vi "SV TDMS Write Spectrum (1 Ch).vi"(0 "tdms file":refnum<k34>, 2 "write mode":u16(ring)=1 items=["Append", "New group", "Overwrite"], 5 "group name in":string="Spectrum", 7 "channel name in":string="Channel0", 9 "spectrum":cluster{"x0":dbl, "dx":dbl, "array":dbl[]}, 11 "error in":errorcluster, 12 "component":T1=32 items=["Magnitude"=32, "Phase"=33, "Real"=34, "Imaginary"=35, "Coherence"=36, "Unknown"=99], 13 "spectrum info":T2 {"x-axis units" items=["Time (s)"=0, "Frequency-CB (Hz)"=1, "Frequency-CPB (Hz)"=1248, "Frequency-Arbitrary (Hz)"=2357, "Quefrency (s)"=2, "Revolutions (rev)"=3, "Order"=4, "Speed (RPM)"=11, "Speed (rad/s)"=21, "Index"=65535]; "weighting filter" items=["Linear", "A-weighting", "B-weighting", "C-weighting", "ITU-R 468-4", "Dolby", "CCITT", "C-message", "Wb", "Wc", "Wd", "We", "Wf", "Wh", "Wj", "Wk", "Wm", "AES17 20 kHz lowpass", "AES17 40 kHz lowpass", "AES17 20 kHz highpass", "AES17 40 kHz highpass"]; "dB reference [EU]" format="%.2f"; "engineering units" items=["custom..."=0, "V"=1, "A"=21, "C"=30, "pC"=31, "s"=32, "-"=29, "Pa"=2, "N"=20, "g"=3, "m/s^2"=4, "m/s"=5, "m"=6, "mm/s"=12, "mm"=13, "micron/s"=14, "micron"=15, "in/s^2"=7, "in/s"=8, "in"=9, "mil/s"=10, "mil"=11, "rad/s^2"=16, "rad/s"=17, "rad"=18, "deg/s^2"=26, "deg/s"=27, "deg"=28, "RPM"=22, "cycle/s^2"=23, "Hz"=24, "cycle"=25, "strain"=19]; "spectral info"."window" items=["None "=0, "Hanning"=1, "Hamming"=2, "Blackman-Harris"=3, "Exact Blackman"=4, "Blackman"=5, "Flat Top"=6, "4 Term B-Harris "=7, "7 Term B-Harris"=8, "Low Sidelobe"=9, "Force - Exponential"=10, "Gaussian"=62]}) -> (4 "tdms file out":refnum<k34>, 6 "group name out":string, 8 "channel name out":string, 15 "error out":errorcluster)   [LabVIEW 2017]
doc: "Writes data to the specified .tdms file in a format specific to the polymorphic instance. Wire data to the <B>scaled signal [EU]</B> input to determine the polymorphic instance to use or manually select the instance."
uses:
  <vilib>/addons/_NISVFA/_Shared subVIs/Controls/svc_Spectrum Info.ctl
  <vilib>/addons/_NISVFA/_Shared subVIs/Controls/svc_X-Axis Units.ctl
  <vilib>/addons/_NISVFA/_Shared subVIs/Controls/svc_Spectrum Type.ctl
  <vilib>/addons/_NISVFA/_Shared subVIs/Controls/svc_Engineering Units Text Ring.ctl
  <vilib>/addons/_NISVFA/_Shared subVIs/Controls/svc_Weighting Filter Text Ring.ctl
  <vilib>/addons/_NISVFA/_Shared subVIs/Controls/svc_Complimentary Spectrum Units.ctl
  <vilib>/addons/_NISVFA/_Shared subVIs/Controls/NI Spectrum Component.ctl
  <vilib>/addons/_NISVFA/_Shared subVIs/Controls/LV Datatypes.ctl
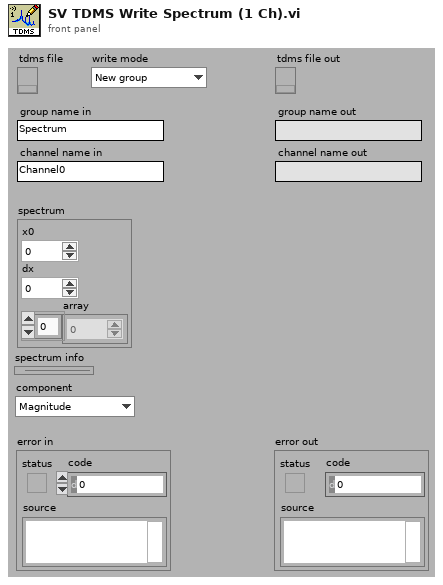
[diagram p1: front panel]
types:
  T1 = typedef "NI Spectrum Component.ctl" = u16
  T2 = typedef "svc_Spectrum Info.ctl" = cluster{"channel name":string, "description":string, "x-axis units":T3, "spectral info":cluster{"spectrum type":T4, "linear/dB":enum16{"linear", "dB"}, "window":u16, "window size":i32, "FFT size":i32}, "engineering units":T5, "custom label":string, "dB reference [EU]":dbl, "peak units":enum16{"rms", "peak", "peak-peak"}, "weighting filter":T6, "spectral density?":bool, "unit label":string, "spectrum skewed?":bool, "complimentary spectrum units":T7}
  T3 = typedef "svc_X-Axis Units.ctl" = u16
  T4 = typedef "svc_Spectrum Type.ctl" = enum16{"FFT Spectrum [complex]", "Amplitude [Magnitude]", "Power [Magnitude^2]", "Cross Spectrum [complex]", "Frequency Response [Complex]"}
  T5 = typedef "svc_Engineering Units Text Ring.ctl" = u16
  T6 = typedef "svc_Weighting Filter Text Ring.ctl" = u16
  T7 = typedef "svc_Complimentary Spectrum Units.ctl" = enum16{"none", "radians", "degrees", "cycles", "imaginary"}
  T8 = typedef "LV Datatypes.ctl" = i32
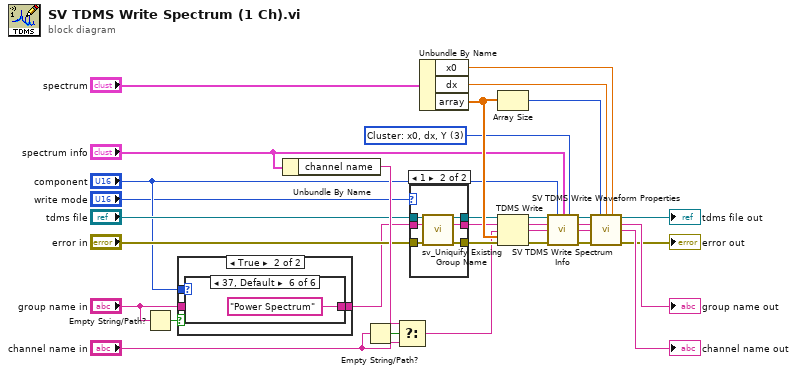
[diagram p0: block diagram]
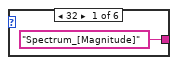
[diagram p4: hidden frame]
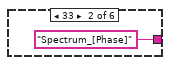
[diagram p5: hidden frame]
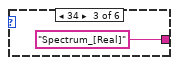
[diagram p6: hidden frame]
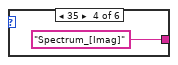
[diagram p7: hidden frame]
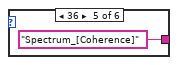
[diagram p8: hidden frame]
diagram:
  w1 = T8 3 items=["String: abc"=-2, "Boolean: True or False"=-1, "Scalar: y"=0, "Array: Y"=1, "Waveform: t0, dt, Y, variant"=2, "Cluster: x0, dx, Y"=3, "Cluster: X, Y"=4, "Waterfall"=5, "Colormap"=6] ("LabVIEW datatype")
  n1 = Empty String/Path?(string/path="group name in") -> (empty?=w21:bool)
  n2 = case shown="True" w21 {
    tunnel: "component" -> [_ w36]
    tunnel: [w34 w35] -> w22
    tunnel: "group name in" -> [w34 _]
    frame False {
    }
    frame True {
      n3 = case shown="37, Default" w36 {
        tunnel: ["Spectrum_[Magnitude]" "Spectrum_[Phase]" "Spectrum_[Real]" "Spectrum_[Imag]" "Spectrum_[Coherence]" "Power Spectrum"] -> w35
        frame 32 {
        }
        frame 33 {
        }
        frame 34 {
        }
        frame 35 {
        }
        frame 36 {
        }
        frame 37, Default {
        }
      }
    }
  }
  n4 = Unbundle By Name("spectrum info") -> ("channel name"=w31:string)
  n5 = Empty String/Path?(string/path="channel name in") -> (empty?=w28:bool)
  n6 = Select(t=w31, s=w28, f="channel name in") -> (s? t:f=w30:string)
  n7 = case shown="1" "write mode" {
    tunnel: [w43 w51] -> w32
    tunnel: [w44 w50] -> w26
    tunnel: "error in" -> [w43 w49]
    tunnel: [w45 w48] -> w23
    tunnel: w22 -> [w44 w47]
    tunnel: "tdms file" -> [w45 w46]
    frame 0, Default {
    }
    frame 1 {
      n8 = call <vilib>:"sv_Uniquify Existing Group Name.vi"("tdms file ref"=w46, "group name"=w47, "error in"=w49) -> ("tdms file out"=w48:refnum<k34>, "unique group"=w50:string, "error out"=w51:errorcluster)  [unwired: 10 in]
    }
  }
  n9 = Unbundle By Name("spectrum") -> ("x0"=w15:dbl, "dx"=w16:dbl, "array"=w33:dbl[])
  n10 = Array Size(array=w33) -> (size(s)=w17:i32)
  n11 = TDMS Write(0:w23, 5:w26, 7:w30, 9:w33, 11:w32) -> (4:w10:refnum<k34>, 6:w9:string, 8:w8:string, 15:w7:errorcluster)  [unwired: 1 in]
  n12 = call <vilib>:"SV TDMS Write Spectrum Info.vi"("tdms file"=w10, "spectrum component"="component", "spectrum info"="spectrum info", "LabVIEW datatype"=w1, "group name in"=w9, "channel name in"=w8, "error in"=w7) -> ("tdms file out"=w11:refnum<k34>, "group name out"=w12:string, "channel name out"=w13:string, "error out"=w14:errorcluster)  [unwired: 3 in, 2 out]
  n13 = call <vilib>:"SV TDMS Write Waveform Properties.vi"("tdms file"=w11, "array length"=w17, "dx"=w16, "x0"=w15, "group name"=w12, "channel name"=w13, "error in (no error)"=w14) -> ("tdms file out"=→"tdms file out":refnum<k34>, "group name out"=→"group name out":string, "channel name out"=→"channel name out":string, "error out"=→"error out":errorcluster)  [unwired: 5 in]
